vi "circulo.vi"() -> ()   [LabVIEW 2020]
panel:
  out "Grafico  de un circulo":cluster{dbl[], dbl[]}(graph)
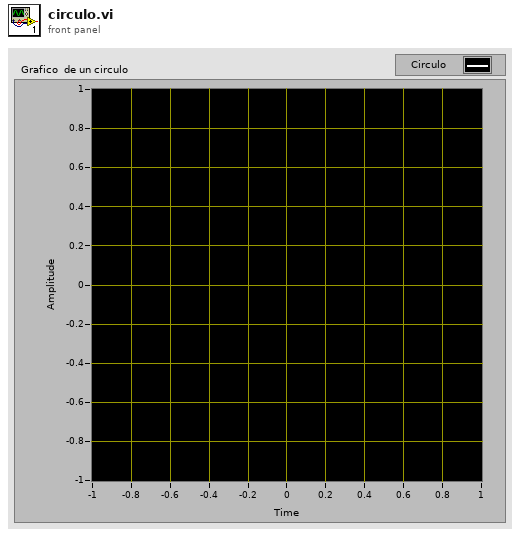
[diagram p1: front panel]
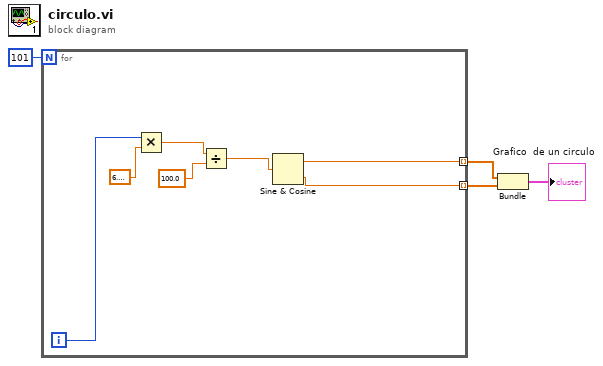
[diagram p0: block diagram]
diagram:
  n1 = for {
    N: 101 -> [_]
    tunnel: [w8] -> w3 mode=indexing
    tunnel: [w7] -> w2 mode=indexing
    i -> [w11]
    n2 = Multiply(x=w11, y=6.283185307179586) -> (x*y=w10:dbl)
    n3 = Divide(x=w10, y=100.0) -> (x/y=w9:dbl)
    n4 = Sine & Cosine(0:w9) -> (1:w8:dbl, 2:w7:dbl)
  }
  n5 = Bundle(w3, w2) -> (→"Grafico  de un circulo":cluster{dbl[], dbl[]})  [unwired: 1 in]
